vi "dfd_Convert Numeric Array to String.vi"(5 "indent order":i32, 6 "display in one line?":bool, 7 "format string":string="%-+024.16e", 11 "numeric array":dbl[](array[numeric])) -> (3 "string":string)   [LabVIEW 2017, in "NI_DigFilter_Process.lvlib"]
uses:
  <vilib>/addons/Digital Filter Design/NI_DigFilter_Process.lvlib
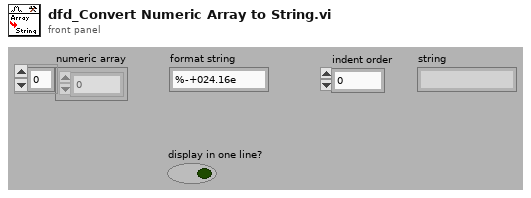
[diagram p1: front panel]
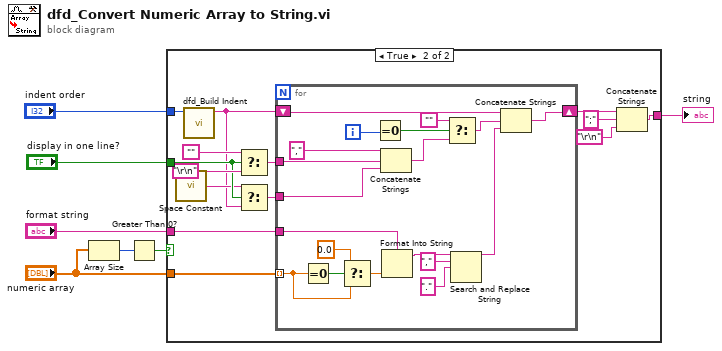
[diagram p0: block diagram]
diagram:
  n1 = Array Size(array="numeric array") -> (size(s)=w2:i32)
  n2 = Greater Than 0?(x=w2) -> (x > 0?=w3:bool)
  n3 = case shown="True" w3 {
    tunnel: "numeric array" -> [_ w21]
    tunnel: "format string" -> [_ w20]
    tunnel: "indent order" -> [_ w16]
    tunnel: [_ w18] -> w5
    tunnel: "display in one line?" -> [_ w11]
    frame False {
    }
    frame True {
      n4 = call <vilib>:"Space Constant.vi"() -> ("String"=w10:string)
      n5 = call <vilib>:"dfd_Build Indent.vi"("indent order"=w16) -> ("tag indent"=w8:string)  [unwired: 10 out]
      n6 = Select(t="", s=w11, f="\r\n") -> (s? t:f=w13:string)
      n7 = Select(t=w10, s=w11, f=w8) -> (s? t:f=w9:string)
      n8 = for {
        tunnel: w21 -> [w22] mode=indexing
        shift-right: [w39] -> w19
        shift-left: w8 -> [w38]
        tunnel: w20 -> [w35]
        tunnel: w13 -> [w34]
        tunnel: w9 -> [w31]
        i -> [w40]
        n9 = Equal To 0?(x=w22) -> (x = 0?=w25:bool)
        n10 = Select(t=0.0, s=w25, f=w22) -> (s? t:f=w24:dbl)
        n11 = Equal To 0?(x=w40) -> (x = 0?=w32:bool)
        n12 = Concatenate Strings(",", w34, w31) -> (w33:string)
        n13 = Format Into String(format string=w35, w24) -> (resulting string=w29:string)  [unwired: 2 in, 1 out]
        n14 = Select(t="", s=w32, f=w33) -> (s? t:f=w37:string)
        n15 = Search and Replace String(input string=w29, search string=",", replace string="." ("replace string (\"\")")) -> (result string=w28:string)  [unwired: 2 in, 6 out]
        n16 = Concatenate Strings(w38, w37, w28) -> (w39:string)
      }
      n17 = Concatenate Strings(w19, ";" ("string"), "\r\n") -> (w18:string)
    }
  }
  "string" <- w5
